vi "improvedUnitsConversion.vi"(10 "Units":string, 11 "Time":dbl) -> (2 "Numeric":dbl)   [LabVIEW 2013]
doc: "Converts a input time given by a number and a string (s, ms, us, ns) into a time in seconds. \nThe number is mutiplied by 10^-0, 10^-3, 10^-6, 10^-9."
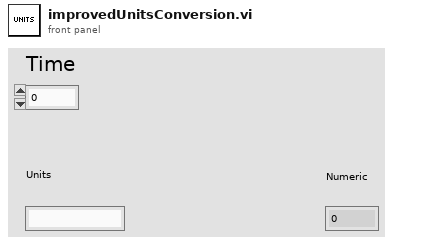
[diagram p1: front panel]
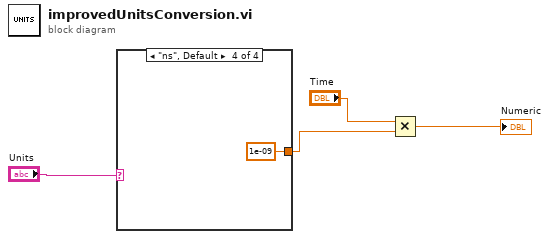
[diagram p0: block diagram]
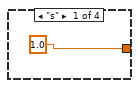
[diagram p2: hidden frame]
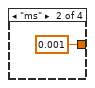
[diagram p3: hidden frame]
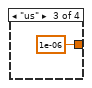
[diagram p4: hidden frame]
diagram:
  n1 = case shown="\"ns\", Default" "Units" {
    tunnel: [1.0 0.001 1e-06 1e-09] -> w3
    frame "s" {
    }
    frame "ms" {
    }
    frame "us" {
    }
    frame "ns", Default {
    }
  }
  n2 = Multiply(x="Time", y=w3) -> (x*y=→"Numeric":dbl)
